vi "CalcHiPressVolt.vi"(0 "Setpoint HI Press":dbl) -> (4 "Numeric":dbl)   [LabVIEW 2019, in "Stand.lvclass"]
uses:
  Stand.lvclass
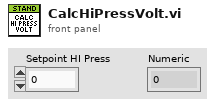
[diagram p1: front panel]
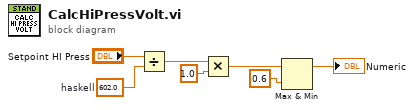
[diagram p0: block diagram]
diagram:
  w5 = 602.0  # haskell
  n1 = Divide(x="Setpoint HI Press", y=w5) -> (x/y=w6:dbl)
  n2 = Multiply(x=w6, y=1.0) -> (x*y=w3:dbl)
  n3 = Max & Min(x=w3, y=0.6) -> (max(x,y)=→"Numeric":dbl)  [unwired: 1 out]
